vi "CR-表面检测图像获取.vi"(1 "数值":dbl, 11 "error in (no error)":errorcluster caption="错误输入（无错误）") -> (4 "iamge4":T1(plugin-control), 6 "iamge5":T1(plugin-control), 10 "iamge3":T1(plugin-control), 15 "error out":errorcluster caption="错误输出")   [LabVIEW 2017]
uses:
  Global System.vi
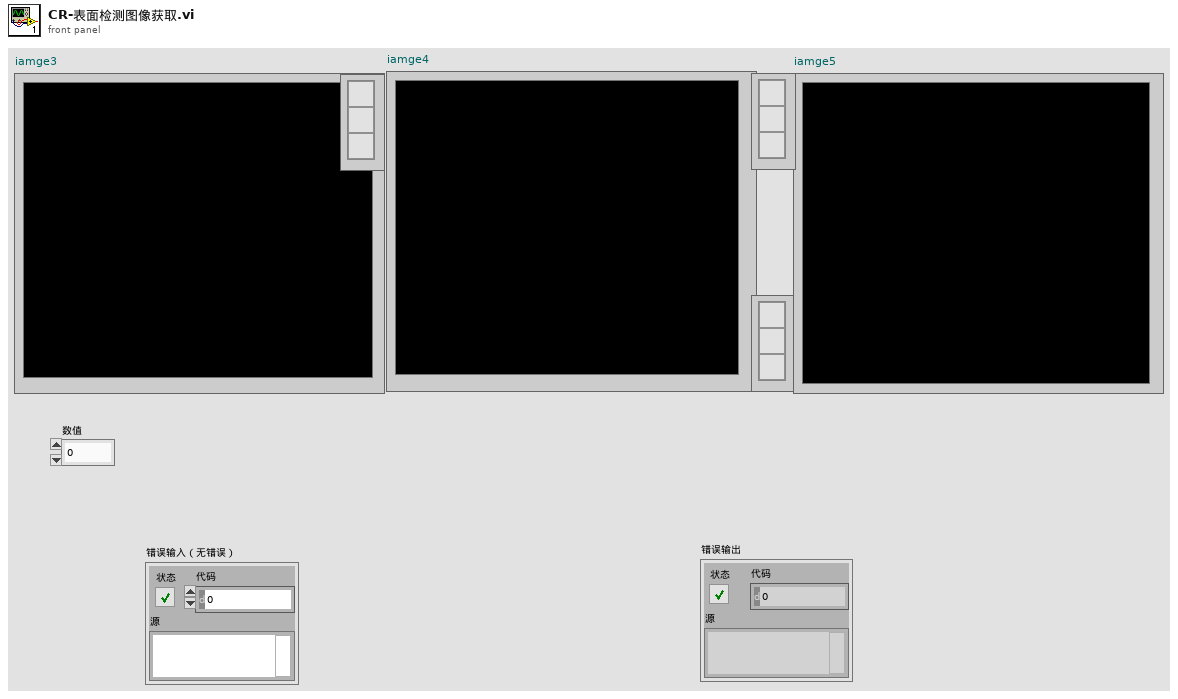
[diagram p1: front panel]
types:
  T1 = typedef "IMAQ Image.ctl" = refnum<image>
  T2 = cluster{"Desired Font (Application)":enum16{"User-specified Font", "Application Font", "System Font", "Dialog Font"}, "[User-specified Font]":cluster{"Font Name":string, "Size":i16, "Strikeout?":bool, "Italic?":bool, "Underline?":bool, "Outline?":bool, "Shadow?":bool, "Bold?":bool, "Rotation Angle":dbl}, "Horizontal Alignment":i16, "Vertical Alignment":i16}
  T3 = typedef "IMAQdx.ctl" = refnum<k21>
  T4 = cluster{"IsNorImage":bool, "Exposure Values":u32, "ImagePath":path, "相机选择":T3}
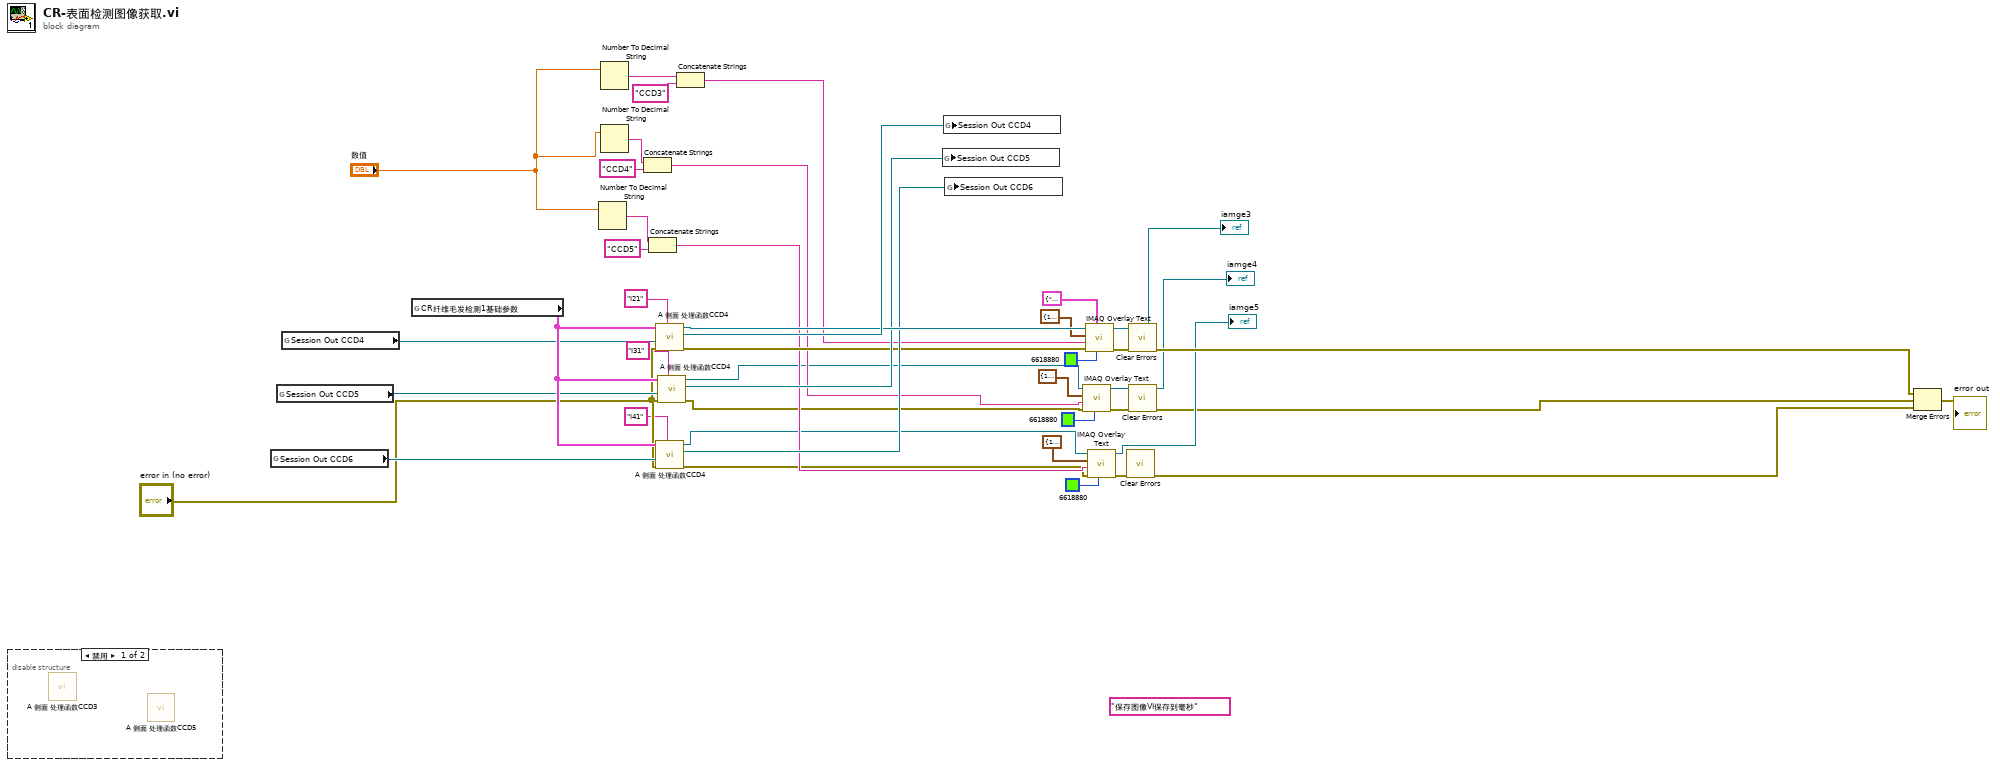
[diagram p0: block diagram]
diagram:
  (unwired) "保存图像VI保存到毫秒"
  n1 = disable-structure shown="禁用" {
    frame Disabled {
      n2 = call "A 侧面 处理函数CCD3.vi"() -> ()  [unwired: 8 in, 4 out]
      n3 = call "A 侧面 处理函数CCD5.vi"() -> ()  [unwired: 8 in, 4 out]
    }
    frame Enabled {
    }
  }
  n4 = global read "Global System.vi" "Session Out CCD6"() -> (w38:T3)
  n5 = global read "Global System.vi" "Session Out CCD5"() -> (w37:T3)
  n6 = global read "Global System.vi" "Session Out CCD4"() -> (w39:T3)
  n7 = global read "Global System.vi" "CR纤维毛发检测1基础参数"() -> (w40:T4)
  n8 = Number To Decimal String(number="数值") -> (decimal integer string=w11:string)  [unwired: 1 in]
  n9 = Number To Decimal String(number="数值") -> (decimal integer string=w34:string)  [unwired: 1 in]
  n10 = Number To Decimal String(number="数值") -> (decimal integer string=w9:string)  [unwired: 1 in]
  n11 = Concatenate Strings(w9, "CCD4" ("字符串")) -> (w10:string)
  n12 = Concatenate Strings(w11, "CCD5" ("字符串")) -> (w12:string)
  n13 = call "A 侧面 处理函数CCD4.vi"("Image Name"="I21", "error in (no error)"="error in (no error)", "相机选择"=w39, "ParamsUI"=w40) -> ("error out"=w22:errorcluster, "Session Out"=w44:T3, "Image out"=w42:T1)  [unwired: 4 in, 1 out]
  n14 = call "A 侧面 处理函数CCD4.vi"("Image Name"="I41", "error in (no error)"="error in (no error)", "相机选择"=w38, "ParamsUI"=w40) -> ("error out"=w4:errorcluster, "Session Out"=w31:T3, "Image out"=w6:T1)  [unwired: 4 in, 1 out]
  n15 = call "A 侧面 处理函数CCD4.vi"("Image Name"="I31", "error in (no error)"="error in (no error)", "相机选择"=w37, "ParamsUI"=w40) -> ("error out"=w5:errorcluster, "Session Out"=w30:T3, "Image out"=w7:T1)  [unwired: 4 in, 1 out]
  n16 = Concatenate Strings(w34, "CCD3" ("字符串")) -> (w16:string)
  n17 = global write "Global System.vi" "Session Out CCD5"(w30) -> ()
  n18 = global write "Global System.vi" "Session Out CCD4"(w44) -> ()
  n19 = global write "Global System.vi" "Session Out CCD6"(w31) -> ()
  n20 = call "IMAQ Overlay Text"("Text Color (black)"=u32 6618880, "error in (no error)"=w5, "String"=w10, "Origin"=cluster{"X":i32, "Y":i32} {"X"=100, "Y"=300}, "Image"=w7) -> ("error out"=w20:errorcluster, "Image Out"=→"iamge4":T1)  [unwired: 5 in]
  n21 = call "IMAQ Overlay Text"("Text Color (black)"=u32 6618880, "Font, Size & Style"=T2 {"Desired Font (Application)"=enum."Application Font", "[User-specified Font]"={"Font Name"="", "Size"=24, "Strikeout?"=FALSE, "Italic?"=FALSE, "Underline?"=FALSE, "Outline?"=FALSE, "Shadow?"=FALSE, "Bold?"=FALSE, "Rotation Angle"=0.0}, "Horizontal Alignment"=0, "Vertical Alignment"=0}, "error in (no error)"=w22, "String"=w16, "Origin"=cluster{"X":i32, "Y":i32} {"X"=100, "Y"=300}, "Image"=w42) -> ("error out"=w21:errorcluster, "Image Out"=→"iamge3":T1)  [unwired: 4 in]
  n22 = call "IMAQ Overlay Text"("Text Color (black)"=u32 6618880, "error in (no error)"=w4, "String"=w12, "Origin"=cluster{"X":i32, "Y":i32} {"X"=100, "Y"=300}, "Image"=w6) -> ("error out"=w19:errorcluster, "Image Out"=→"iamge5":T1)  [unwired: 5 in]
  n23 = call <vilib>:"Clear Errors.vi"("error in (no error)"=w19) -> ("error out"=w17:errorcluster)  [unwired: 5 in, 1 out]
  n24 = call <vilib>:"Clear Errors.vi"("error in (no error)"=w21) -> ("error out"=w43:errorcluster)  [unwired: 5 in, 1 out]
  n25 = call <vilib>:"Clear Errors.vi"("error in (no error)"=w20) -> ("error out"=w18:errorcluster)  [unwired: 5 in, 1 out]
  n26 = Merge Errors(w43, w18, w17) -> (→"error out":errorcluster)
